vi "Get Data Version.vi"(8 "error in":errorcluster, 11 "RDMA Rx Transfer Configuration in":refnum<class "RDMA Transfer Rx Configuration.lvclass">) -> (0 "error out":errorcluster, 2 "data version":T1, 3 "RDMA Rx Transfer Configuration out":refnum<class "RDMA Transfer Rx Configuration.lvclass">)   [LabVIEW 2020, in "RDMA.lvlib" / "RDMA Transfer Rx Configuration.lvclass"]
uses:
  RDMA Transfer Rx Configuration.lvclass
  DSF Core.lvlibp/Typedefs/DSF Version Info.ctl
  DSF Core.lvlibp
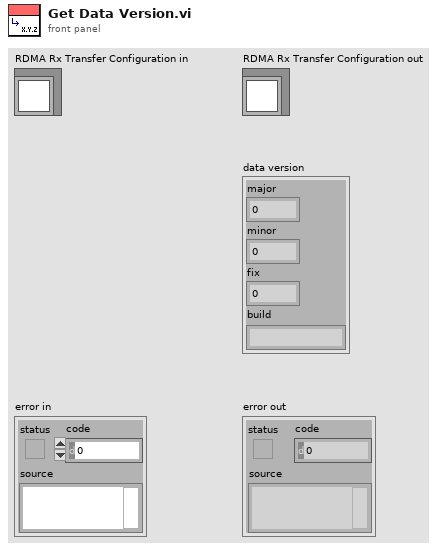
[diagram p1: front panel]
types:
  T1 = typedef "DSF Core.lvlibp/DSF Version Info.ctl" = cluster{"major":u32, "minor":u32, "fix":u32, "build":string}
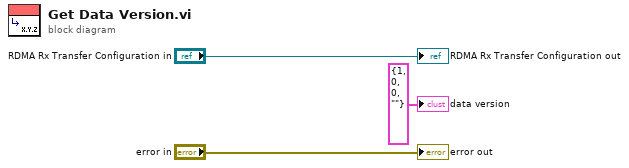
[diagram p0: block diagram]
diagram:
  "error out" <- "error in"
  "RDMA Rx Transfer Configuration out" <- "RDMA Rx Transfer Configuration in"
  "data version" <- T1 {"major"=1, "minor"=0, "fix"=0, "build"=""} ("data version")
